vi "Main.vi"() -> ()   [LabVIEW 2017]
doc: "This Continuous Measurement sample project is based on the Queued Message Handler template.\n\nThe Event Handling Loop generates messages based on user interface actions.\n\nThe Message Handling Loop processes messages generated by the Event Handling Loop, or by other messages. There are also Acquisition and Logging message handling loop subVIs, and a chart updating loop."
uses:
  Settings/Settings.ctl
  Acquisition/Hardware Configuration.ctl
  Acquisition/Signal Type.ctl
  Logging/Logging Configuration.ctl
  controls/UI Data.ctl
  controls/UI State.ctl
  support/Message Queue/Enqueue Message (Single).vi
  support/Message Queue/Enqueue Message (Array).vi
  <vilib>/Utility/error.llb/Error Cluster From Error Code.vi
  <vilib>/ErrorRing/Error Ring.xnode
  Acquisition/Acquisition.lvlib
  Logging/Logging.lvlib
  Settings/Settings.lvlib
  support/User Event - Stop/User Event - Stop.lvlib
  support/Message Queue/Message Queue.lvlib
  Settings/Settings Dialog.vi
panel:
  out "Zero run":bool
  in  "Zero run?":bool
  out "Max writing time to a file [min]":dbl
  out "Elapsed time":timestamp
  out "Test time zero run [s]":dbl
  out "Test time [s]":dbl
  in  "Start":bool
  in  "Stop":bool
  in  "Settings":bool
  out "Status":string
  in  "Exit":bool
  out "Log File Offsite Path":path
  out "Project code":string
  out "Offsite storage?":bool
  out "Log File Path":path
  out "Data":waveform(dbl)[](graph)
  # "Continuous Measurement Data Logger"
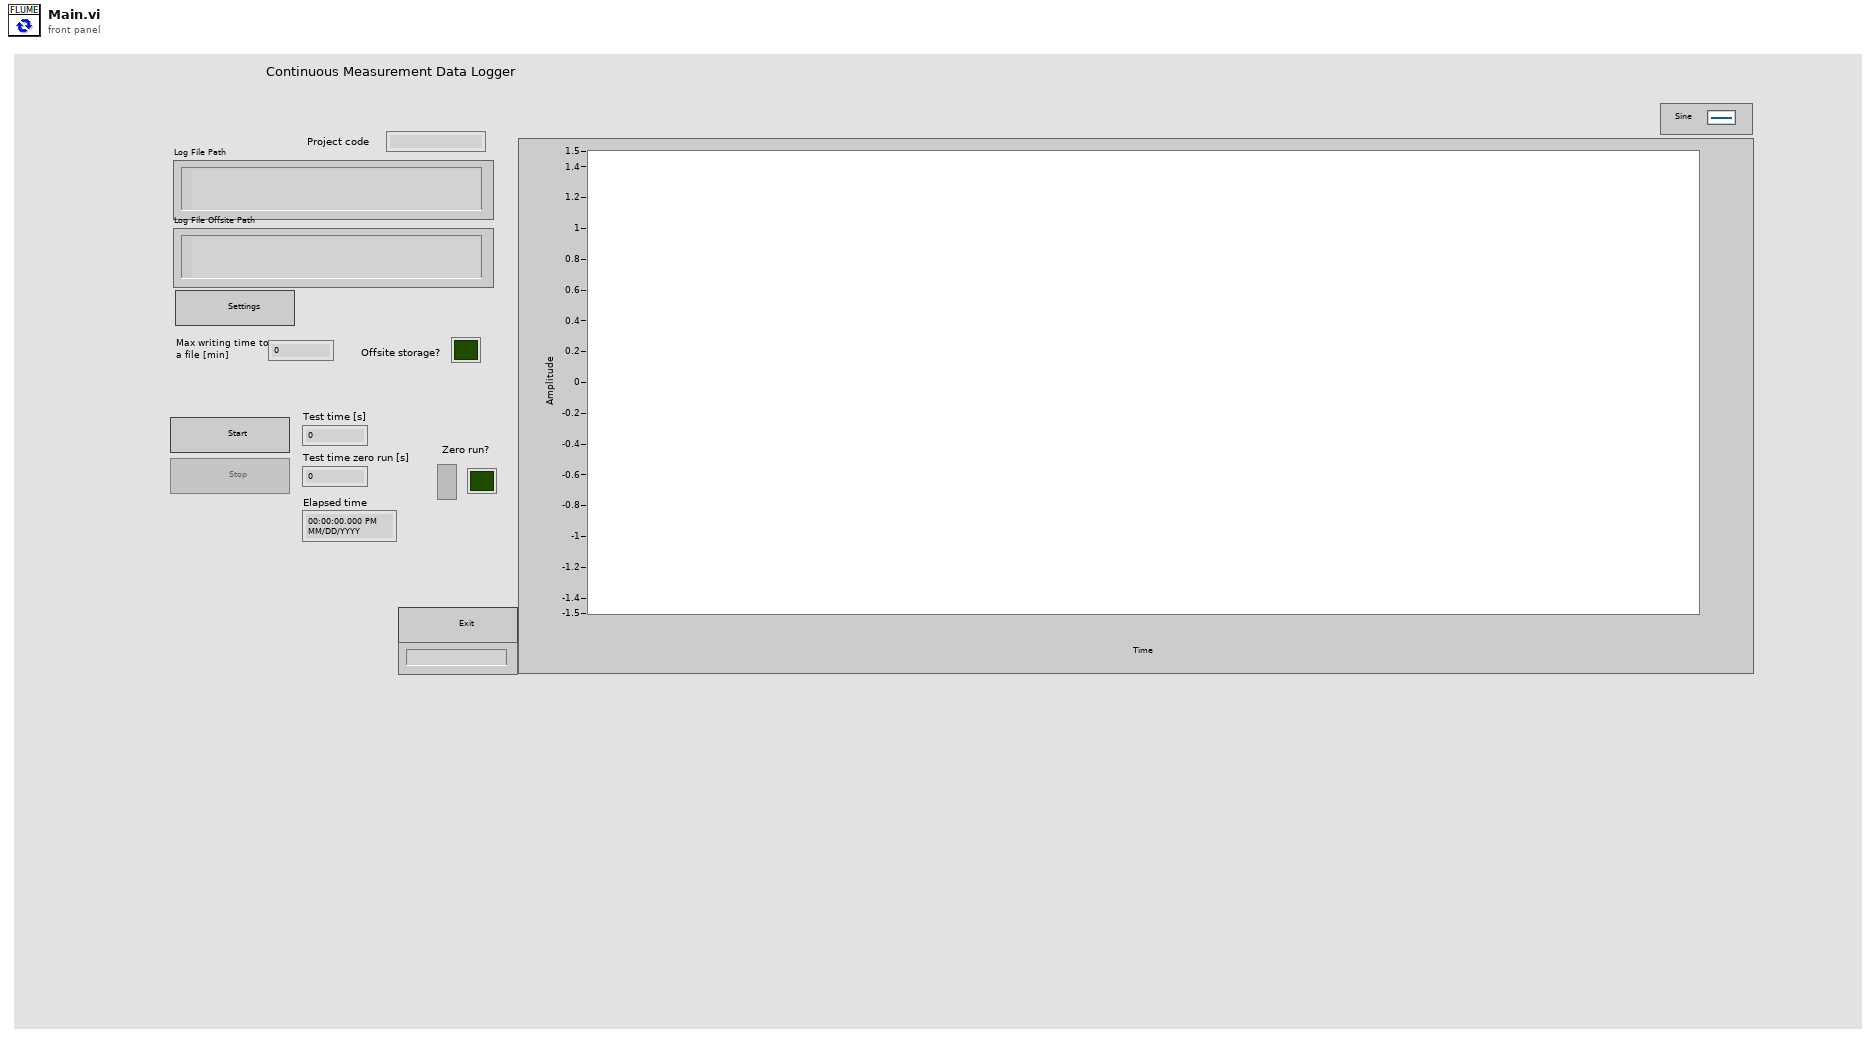
[diagram p1: front panel]
types:
  T1 = cluster{"Offsite storage?":bool, "Test time [s]":dbl, "Test time zero run [s] ":dbl, "Max writing time to a file [min]":dbl, "Zero run":bool}
  T2 = typedef "UI State.ctl" = enum16{"Idle", "Acquiring and Logging", "Waiting for Exit", "Waiting for Exit (Acq Stopped)", "Waiting for Exit (Log Stopped)", "Waiting for Stop", "Waiting for Stop (Acq Stopped)", "Waiting for Stop (Log Stopped)"}
  T3 = typedef "UI Data.ctl" = cluster{"Start Ref":refnum<vi>, "Stop Ref":refnum<vi>, "Settings Ref":refnum<vi>, "Exit Ref":refnum<vi>, "Status Ref":refnum<vi>, "Data Ref":refnum<vi>, "Zero run Ref":refnum<vi>}
  T4 = typedef "Settings.lvlib/Settings.ctl" = cluster{"Hardware Configuration":T5, "Logging Configuration":T7, "Timers":cluster{"Offsite storage?":bool, "Test time [s]":dbl, "Test time zero run [s] ":dbl, "Max writing time to a file [min]":dbl, "Zero run":bool}}
  T5 = typedef "Acquisition.lvlib/Hardware Configuration.ctl" = cluster{"HW Refnum <Replace Me>":string, "Signal Type <Replace Me>":T6}
  T6 = typedef "Acquisition.lvlib/Signal Type.ctl" = enum16{"Sine Wave", "Square with Noise"}
  T7 = typedef "Logging.lvlib/Logging Configuration.ctl" = cluster{"Log File Base Path":path, "TDMS File Reference":refnum<k34>, "Log File Offsite Path":path, "Project code":string, "Bin File Reference":refnum<file>}
  T8 = typedef "Message Queue.lvlib/All Message Queues.ctl" = cluster{"UI":refnum<queue>, "Acquisition":refnum<queue>, "Logging":refnum<queue>, "Bin Logging":refnum<queue>, "Time":refnum<queue>}
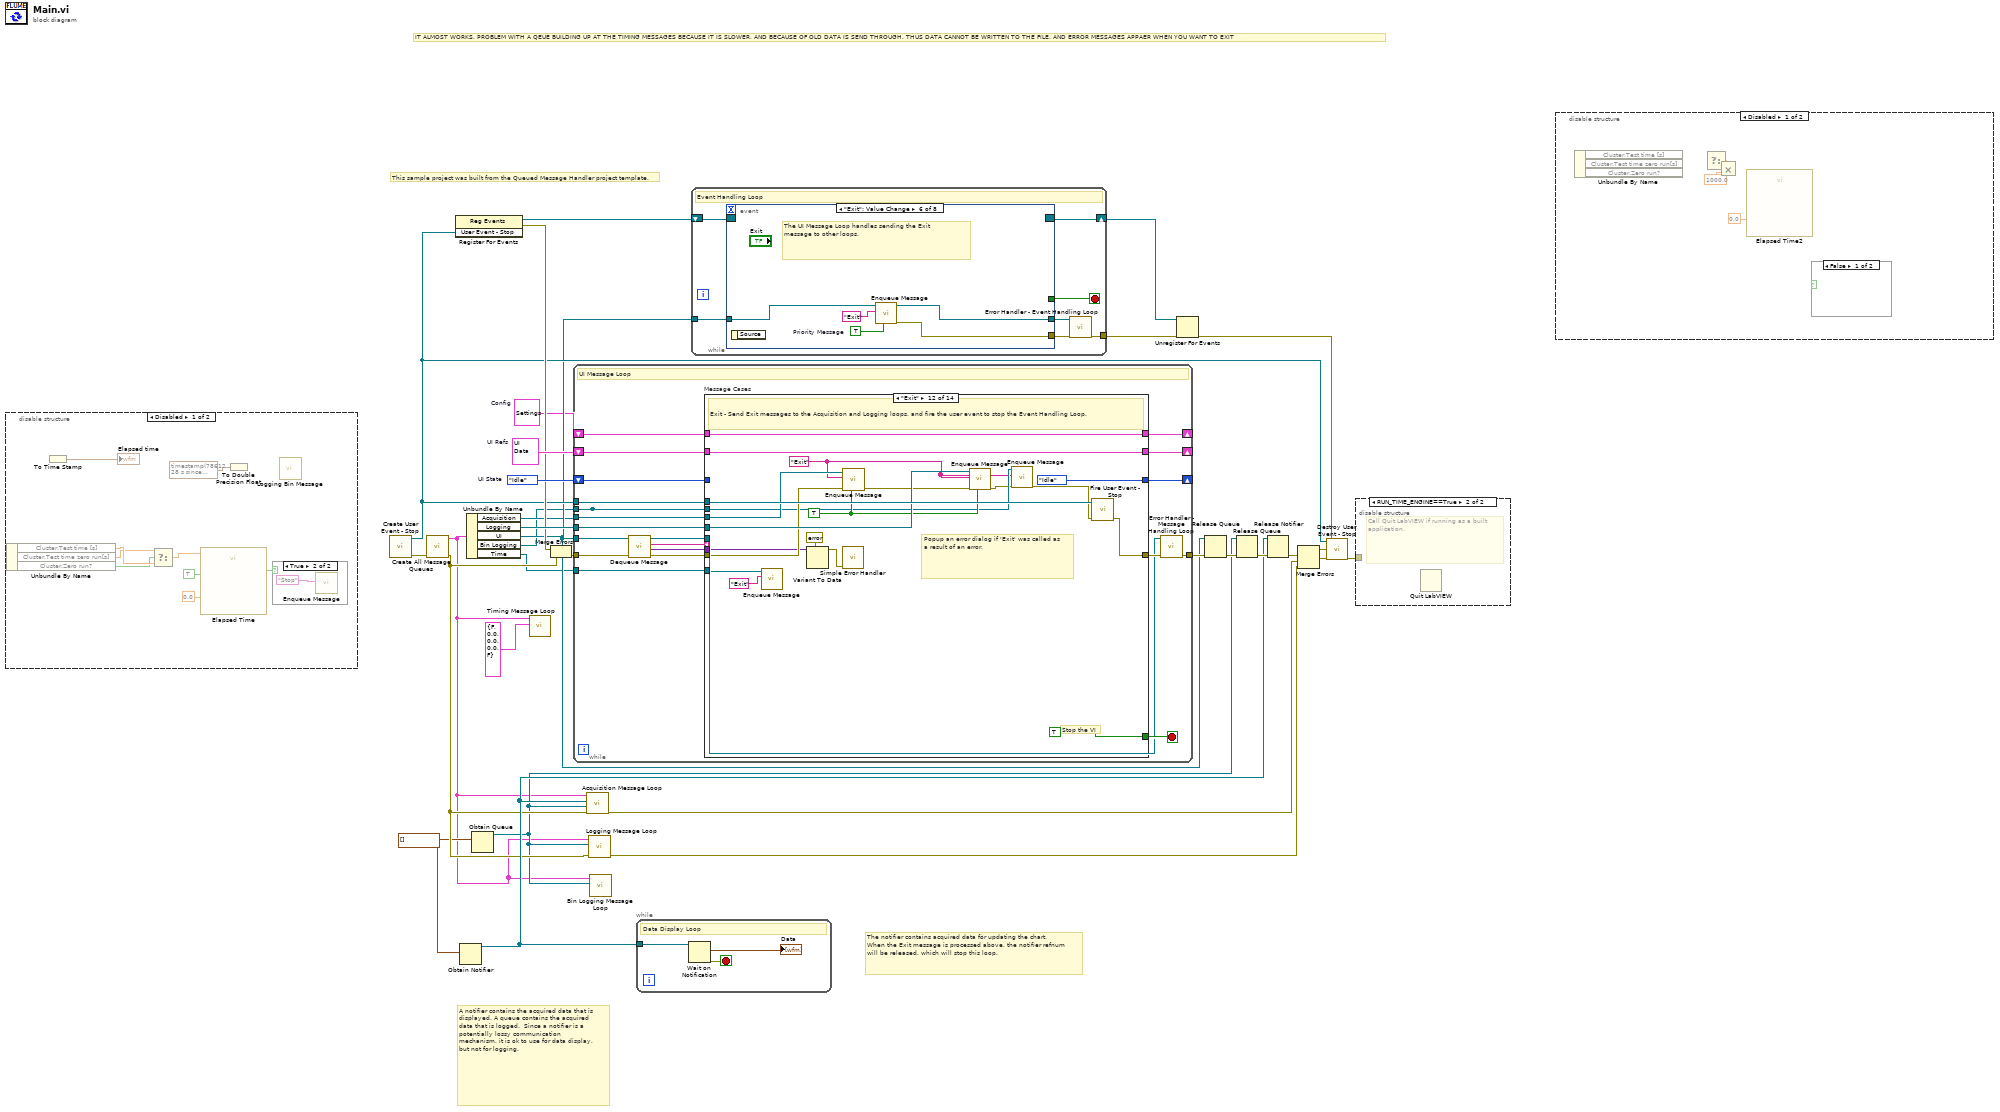
[diagram p0: block diagram]
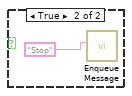
[diagram p2: hidden frame]
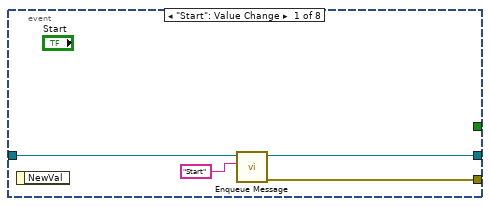
[diagram p7: hidden frame]
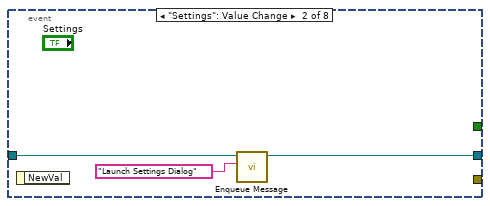
[diagram p8: hidden frame]
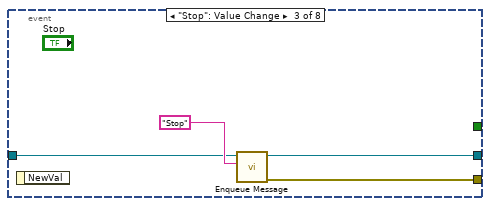
[diagram p9: hidden frame]
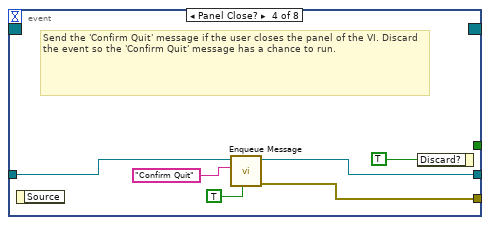
[diagram p10: hidden frame]
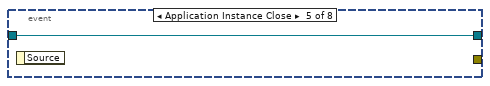
[diagram p11: hidden frame]
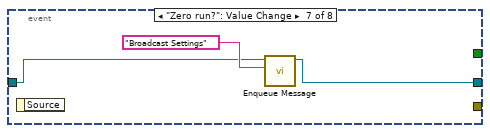
[diagram p12: hidden frame]
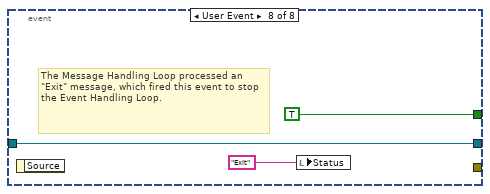
[diagram p13: hidden frame]
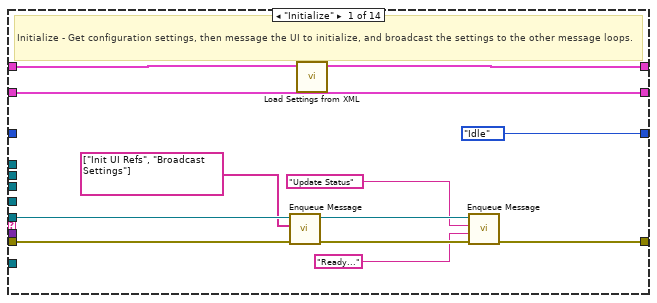
[diagram p14: hidden frame]
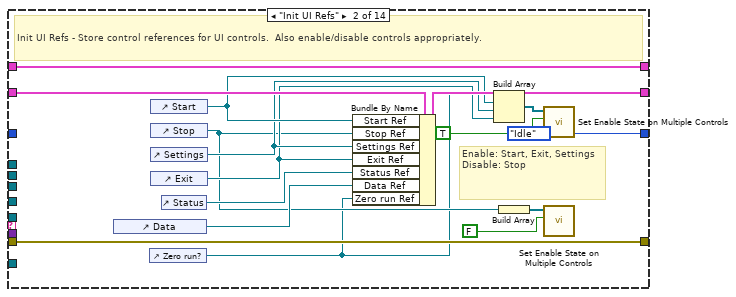
[diagram p15: hidden frame]
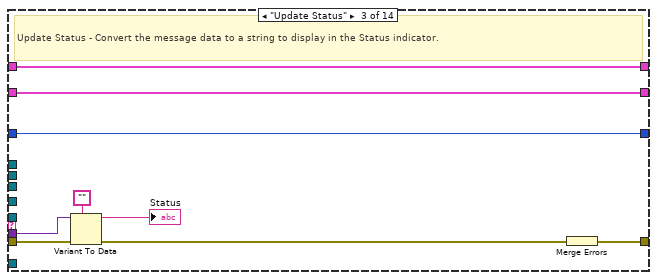
[diagram p16: hidden frame]
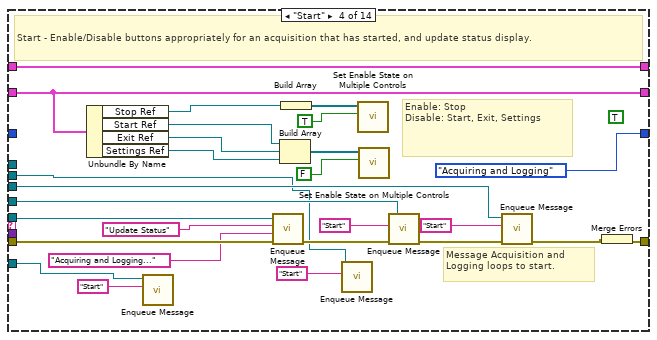
[diagram p17: hidden frame]
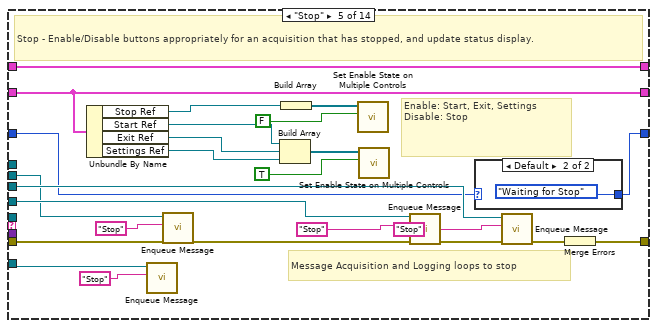
[diagram p18: hidden frame]
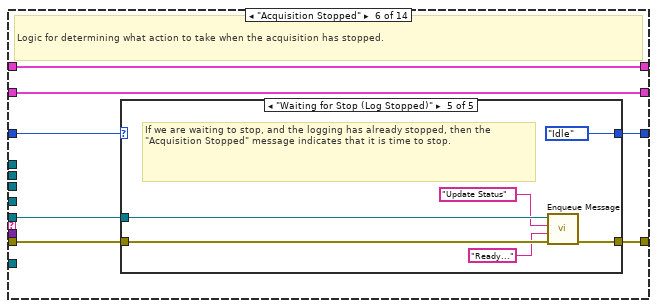
[diagram p20: hidden frame]
diagram:
  w23 = UI_State."Idle"  # UI State
  w7 = waveform(dbl)[] []
  w25 = T3 {"Start Ref"=refnum, "Stop Ref"=refnum, "Settings Ref"=refnum, "Exit Ref"=refnum, "Status Ref"=refnum, "Data Ref"=refnum, "Zero run Ref"=refnum}  # UI Refs
  w9 = T4 {"Hardware Configuration"={"HW Refnum <Replace Me>"="", "Signal Type <Replace Me>"=enum."Sine Wave"}, "Logging Configuration"={"Log File Base Path"=path "", "TDMS File Reference"=refnum, "Log File Offsite Path"=path "", "Project code"="", "Bin File Reference"=refnum}, "Timers"={"Offsite storage?"=FALSE, "Test time [s]"=10.0, "Test time zero run [s] "=180.0, "Max writing time to a file [min]"=30.0, "Zero run"=FALSE}}  # Config
  # "IT ALMOST WORKS, PROBLEM WITH A QEUE BUILDING UP AT THE TIMING MESSAGES BECAUSE IT IS SLOWER, AND BECAUSE OF OLD DATA IS SEND THROUGH, THUS DATA CANNOT BE WRITTEN TO THE FILE, AND ERROR MESSAGES APPAER WHEN YOU WANT TO EXIT"
  # "This sample project was built from the Queued Message Handler project template."
  # "A notifier contains the acquired data that is displayed. A queue contains the acquired data that is logged.  Since a notifier is a potentially lossy communication mechanism, it is ok to use for data display, but not for logging."
  # "The notifier contains acquired data for updating the chart. When the Exit message is processed above, the notifier refnum will be released, which will stop this loop."
  n1 = disable-structure shown="Disabled" {
    frame Disabled {
      n2 = Unbundle By Name() -> ("Cluster.Test time [s]"=w37:dbl, "Cluster.Test time zero run[s]"=w35:dbl, "Cluster.Zero run?"=w34:bool)  [unwired: 1 in]
      n3 = To Time Stamp() -> (0:→"Elapsed time":timestamp)  [unwired: 1 in]
      n4 = Select(t=w35, s=w34, f=w37) -> (s? t:f=w36:dbl)
      n5 = call "Elapsed Time"("Time Target (s)"=w36, "Auto Reset"=TRUE, "Set Start Time (s)"=0.0) -> ("Time has Elapsed"=w33:bool)  [unwired: 9 in, 7 out]
      n6 = To Double Precision Float(number=timestamp(7861228 s since 1904-01-01)) -> ()  [unwired: 1 out]
      n7 = case shown="True" w33 {
        frame False {
        }
        frame True {
          n8 = call-poly "Enqueue Message.vi"("Message"="Stop") -> ()  [unwired: 9 in, 2 out]
        }
      }
      n9 = call "Logging Bin Message.vi"() -> ()  [unwired: 11 in, 1 out]
    }
    frame Enabled {
    }
  }
  n10 = call "Create User Event - Stop.vi"() -> ("error out"=w27:errorcluster, "User Event - Stop"=w14:refnum<user-event>)  [unwired: 10 in]
  n11 = call "Create All Message Queues.vi"("error in (no error)"=w27) -> ("error out"=w8:errorcluster, "Message Queues out"=w2:T8)  [unwired: 9 in]
  n12 = register-events(w14) -> (reference out=w17:refnum<event-registration>, error out=w15:errorcluster)  [unwired: 2 in]
  n13 = Obtain Notifier(notification data type=w7) -> (notifier out=w10:refnum<notifier>)  [unwired: 3 in, 2 out]
  n14 = Unbundle By Name(w2) -> ("Acquisition"=w12:refnum<queue>, "Logging"=w24:refnum<queue>, "UI"=w13:refnum<queue>, "Bin Logging"=w5:refnum<queue>, "Time"=w1:refnum<queue>)
  n15 = Obtain Queue(element data type=w7) -> (queue out=w6:refnum<queue>)  [unwired: 4 in, 2 out]
  n16 = call "Timing Message Loop.vi"("Timers"=T1 {"Offsite storage?"=FALSE, "Test time [s]"=0.0, "Test time zero run [s] "=0.0, "Max writing time to a file [min]"=0.0, "Zero run"=FALSE}, "Message Queues"=w2) -> ()  [unwired: 9 in, 1 out]
  n17 = Merge Errors(w15, w8) -> (w16:errorcluster)
  n18 = while {
    tunnel: w13 -> [w46]
    tunnel: w14 -> [w59]
    shift-right: [w54] -> _
    shift-left: w9 -> [w42]
    shift-right: [w52] -> _
    shift-left: w25 -> [w53]
    tunnel: w12 -> [w51]
    tunnel: w24 -> [w45]
    shift-right: [w47] -> _
    shift-left: w23 -> [w48]
    tunnel: w16 -> [w58]
    tunnel: [w50] -> w30
    tunnel: w5 -> [w43]
    tunnel: [w43] -> _
    tunnel: w1 -> [w41]
    stop <- w60 stop-if-true
    # "UI Message Loop"
    n19 = call "Dequeue Message.vi"("error in (no error)"=w58, "Message Queue"=w46) -> ("error out"=w57:errorcluster, "Message Data"=w55:variant, "Message"=w56:string, "dup Message Queue"=w44:refnum<queue>)  [unwired: 6 in]
    n20 = case "Message Cases" shown="\"Exit\"" w56 {
      selector: w56 -> [_ _ _ _ _ _ _ _ _ _ _ _ _ w304]
      tunnel: w44 -> [w65 _ _ w103 _ w154 w179 _ w232 _ w254 _ _ _]
      tunnel: w57 -> [w64 w88 w96 w124 w147 w155 w180 w222 w234 w242 w253 w288 w302 _]
      tunnel: [w69 w88 w97 w105 w148 w152 w177 w226 w228 w245 w252 w295 w301 w303] -> w49
      tunnel: [_ _ _ _ _ _ _ _ _ _ _ TRUE _ _] -> w60
      tunnel: w55 -> [_ _ w95 _ _ _ _ _ _ w246 _ w286 _ _]
      tunnel: w59 -> [_ _ _ _ _ _ _ _ _ _ _ w296 _ _]
      tunnel: [w72 w75 w89 w101 w129 w151 w176 w205 w227 w241 w250 w284 w300 w307] -> w54
      tunnel: w42 -> [w61 w75 w89 w101 w129 w151 w176 w210 w235 w241 w250 w284 w300 w307]
      tunnel: w53 -> [w66 w87 w91 w121 w146 w157 w182 w221 w230 w249 w256 w294 w299 w306]
      tunnel: [w66 w84 w91 w121 w146 w157 w182 w221 w230 w249 w256 w294 w299 w306] -> w52
      tunnel: w51 -> [_ _ _ w104 w133 _ _ w220 _ _ _ w293 _ _]
      tunnel: w45 -> [_ _ _ w110 w136 _ _ w219 _ _ _ w292 _ _]
      tunnel: w48 -> [_ _ w90 _ w130 w156 w181 w218 w229 w244 w255 _ w298 w305]
      tunnel: [UI_State."Idle" ("UI State") UI_State."Idle" ("UI State") w90 UI_State."Acquiring and Logging" ("UI State") w131 w153 w178 w218 w229 w244 w251 UI_State."Idle" ("UI State") w298 w305] -> w47
      tunnel: w43 -> [_ _ _ w100 w127 _ _ w213 _ _ _ w283 _ _]
      tunnel: w41 -> [_ _ _ w98 w126 _ _ w209 _ _ _ w279 _ _]
      frame "Initialize" {
        # "Initialize - Get configuration settings, then message the UI to initialize, and broadcast the settings to the other message loops."
        n21 = call-poly "Enqueue Message.vi"("error in (no error)"=w64, "Message Array"=string[] ["Init UI Refs", "Broadcast Settings"], "Message Queue"=w65) -> ("error out"=w71:errorcluster, "dup Message Queue"=w70:refnum<queue>)  [unwired: 7 in]
        n22 = call "Load Settings from XML.vi"("Settings in"=w61) -> ("Settings out"=w72:T4)  [unwired: 9 in, 1 out]
        n23 = call-poly "Enqueue Message.vi"("error in (no error)"=w71, "Message Data"="Ready..." ("Ready..."), "Message"="Update Status", "Message Queue"=w70) -> ("error out"=w69:errorcluster)  [unwired: 6 in, 1 out]
      }
      frame "Init UI Refs" {
        # "Enable: Start, Exit, Settings\nDisable: Stop"
        # "Init UI Refs - Store control references for UI controls.  Also enable/disable controls appropriately."
        n24 = control-ref of="Data"() -> (w85:refnum<vi>)
        n25 = control-ref of="Zero run?"() -> (w73:refnum<vi>)
        n26 = control-ref of="Start"() -> (w79:refnum<vi>)
        n27 = control-ref of="Stop"() -> (w74:refnum<vi>)
        n28 = control-ref of="Settings"() -> (w78:refnum<vi>)
        n29 = control-ref of="Exit"() -> (w77:refnum<vi>)
        n30 = control-ref of="Status"() -> (w86:refnum<vi>)
        n31 = Bundle By Name(cluster=w87, "Start Ref"=w79, "Stop Ref"=w74, "Settings Ref"=w78, "Exit Ref"=w77, "Status Ref"=w86, "Data Ref"=w85, "Zero run Ref"=w73) -> (w84:T3)
        n32 = Build Array(w73, w79, w78, w77) -> (w82:refnum<vi>[])
        n33 = Build Array(w74) -> (w81:refnum<vi>[])
        n34 = call "Set Enable State on Multiple Controls.vi"("Enable?"=TRUE, "Controls"=w82) -> ()  [unwired: 10 in]
        n35 = call "Set Enable State on Multiple Controls.vi"("Enable?"=FALSE, "Controls"=w81) -> ()  [unwired: 10 in]
      }
      frame "Update Status" {
        # "Update Status - Convert the message data to a string to display in the Status indicator."
        n36 = Variant To Data(error in=w96, type="", Variant=w95) -> (data=→"Status":string, error out=w93:errorcluster)
        n37 = Merge Errors(w93) -> (w97:errorcluster)
      }
      frame "Start" {
        (unwired) TRUE ("Reset")
        # "Message Acquisition and Logging loops to start."
        # "Enable: Stop\nDisable: Start, Exit, Settings"
        # "Start - Enable/Disable buttons appropriately for an acquisition that has started, and update status display."
        n38 = Unbundle By Name(w121) -> ("Stop Ref"=w116:refnum<vi>, "Start Ref"=w115:refnum<vi>, "Exit Ref"=w114:refnum<vi>, "Settings Ref"=w113:refnum<vi>)
        n39 = call-poly "Enqueue Message.vi"("Message"="Start", "Message Queue"=w98) -> ()  [unwired: 8 in, 2 out]
        n40 = call-poly "Enqueue Message.vi"("error in (no error)"=w124, "Message Data"="Acquiring and Logging..." ("Acquiring and Logging..."), "Message"="Update Status", "Message Queue"=w103) -> ("error out"=w112:errorcluster)  [unwired: 6 in, 1 out]
        n41 = Build Array(w115, w114, w113) -> (w119:refnum<vi>[])
        n42 = Build Array(w116) -> (w118:refnum<vi>[])
        n43 = call-poly "Enqueue Message.vi"("Message"="Start", "Message Queue"=w100) -> ()  [unwired: 8 in, 2 out]
        n44 = call "Set Enable State on Multiple Controls.vi"("Enable?"=TRUE, "Controls"=w118) -> ()  [unwired: 10 in]
        n45 = call "Set Enable State on Multiple Controls.vi"("Enable?"=FALSE, "Controls"=w119) -> ()  [unwired: 10 in]
        n46 = call-poly "Enqueue Message.vi"("error in (no error)"=w112, "Message"="Start", "Message Queue"=w110) -> ("error out"=w107:errorcluster)  [unwired: 7 in, 1 out]
        n47 = call-poly "Enqueue Message.vi"("error in (no error)"=w107, "Message"="Start", "Message Queue"=w104) -> ("error out"=w106:errorcluster)  [unwired: 7 in, 1 out]
        n48 = Merge Errors(w106) -> (w105:errorcluster)
      }
      frame "Stop" {
        # "Message Acquisition and Logging loops to stop"
        # "Enable: Start, Exit, Settings\nDisable: Stop"
        # "Stop - Enable/Disable buttons appropriately for an acquisition that has stopped, and update status display."
        n49 = Unbundle By Name(w146) -> ("Stop Ref"=w141:refnum<vi>, "Start Ref"=w140:refnum<vi>, "Exit Ref"=w139:refnum<vi>, "Settings Ref"=w138:refnum<vi>)
        n50 = call-poly "Enqueue Message.vi"("Message"="Stop", "Message Queue"=w126) -> ()  [unwired: 8 in, 2 out]
        n51 = call-poly "Enqueue Message.vi"("Message"="Stop", "Message Queue"=w127) -> ()  [unwired: 8 in, 2 out]
        n52 = Build Array(w140, w139, w138) -> (w144:refnum<vi>[])
        n53 = Build Array(w141) -> (w143:refnum<vi>[])
        n54 = call "Set Enable State on Multiple Controls.vi"("Enable?"=FALSE, "Controls"=w143) -> ()  [unwired: 10 in]
        n55 = call "Set Enable State on Multiple Controls.vi"("Enable?"=TRUE, "Controls"=w144) -> ()  [unwired: 10 in]
        n56 = call-poly "Enqueue Message.vi"("error in (no error)"=w147, "Message"="Stop", "Message Queue"=w136) -> ("error out"=w135:errorcluster)  [unwired: 7 in, 1 out]
        n57 = case shown="Default" w130 {
          selector: w130 -> [w149 _]
          tunnel: [w149 UI_State."Waiting for Stop" ("UI State")] -> w131
          frame "Waiting for Exit" {
          }
          frame Default {
          }
        }
        n58 = call-poly "Enqueue Message.vi"("error in (no error)"=w135, "Message"="Stop", "Message Queue"=w133) -> ("error out"=w134:errorcluster)  [unwired: 7 in, 1 out]
        n59 = Merge Errors(w134) -> (w148:errorcluster)
      }
      frame "Acquisition Stopped" {
        # "Logic for determining what action to take when the acquisition has stopped."
        n60 = case shown="\"Waiting for Stop (Log Stopped)\"" w156 {
          selector: w156 -> [w159 _ _ _ _]
          tunnel: w155 -> [w158 w161 w163 w169 w175]
          tunnel: w154 -> [_ _ _ w167 w172]
          tunnel: [w159 UI_State."Waiting for Exit (Acq Stopped)" ("UI State") UI_State."Waiting for Stop (Acq Stopped)" ("UI State") UI_State."Idle" ("UI State") UI_State."Idle" ("UI State")] -> w153
          tunnel: [w158 w161 w163 w168 w173] -> w152
          frame Default {
          }
          frame "Waiting for Exit", "Waiting for Exit (Acq Stopped)" {
          }
          frame "Waiting for Stop", "Waiting for Stop (Acq Stopped)" {
          }
          frame "Waiting for Exit (Log Stopped)" {
            # "If we are waiting to exit, and the logging has already stopped, then the \"Acquisition Stopped\" message indicates that it is time to exit."
            n61 = call-poly "Enqueue Message.vi"("Priority Message? (F)"=TRUE, "error in (no error)"=w169, "Message"="Exit", "Message Queue"=w167) -> ("error out"=w168:errorcluster)  [unwired: 6 in, 1 out]
          }
          frame "Waiting for Stop (Log Stopped)" {
            # "If we are waiting to stop, and the logging has already stopped, then the \"Acquisition Stopped\" message indicates that it is time to stop."
            n62 = call-poly "Enqueue Message.vi"("error in (no error)"=w175, "Message Data"="Ready..." ("Ready..."), "Message"="Update Status", "Message Queue"=w172) -> ("error out"=w173:errorcluster)  [unwired: 6 in, 1 out]
          }
        }
      }
      frame "Logging Stopped" {
        # "Logic for determining what action to take when the logging has stopped."
        n63 = case shown="Default" w181 {
          selector: w181 -> [w184 _ _ _ _]
          tunnel: w180 -> [w183 w186 w188 w194 w197]
          tunnel: w179 -> [_ _ _ w192 w196]
          tunnel: [w184 UI_State."Waiting for Exit (Log Stopped)" ("UI State") UI_State."Waiting for Stop (Log Stopped)" ("UI State") UI_State."Idle" ("UI State") UI_State."Idle" ("UI State")] -> w178
          tunnel: [w183 w186 w188 w193 w195] -> w177
          frame Default {
          }
          frame "Waiting for Exit", "Waiting for Exit (Log Stopped)" {
          }
          frame "Waiting for Stop", "Waiting for Stop (Log Stopped)" {
          }
          frame "Waiting for Exit (Acq Stopped)" {
            # "If we are waiting to exit, and the acquisition has already stopped, then the \"Logging Stopped\" message indicates that it is time to exit."
            n64 = call-poly "Enqueue Message.vi"("Priority Message? (F)"=TRUE, "error in (no error)"=w194, "Message"="Exit", "Message Queue"=w192) -> ("error out"=w193:errorcluster)  [unwired: 6 in, 1 out]
          }
          frame "Waiting for Stop (Acq Stopped)" {
            # "If we are waiting to stop, and the acquisition has already stopped, then the \"Logging Stopped\" message indicates that it is time to stop."
            n65 = call-poly "Enqueue Message.vi"("error in (no error)"=w197, "Message Data"="Ready..." ("Ready..."), "Message"="Update Status", "Message Queue"=w196) -> ("error out"=w195:errorcluster)  [unwired: 6 in, 1 out]
          }
        }
      }
      frame "Broadcast settings" {
        w208 = "Update Settings" ("Message")
        # "Broadcast settings - Send the 'Update Settings' message to the Logging and Acquisition message loops."
        n66 = Unbundle By Name(w210) -> ("Hardware Configuration"=w224:T5, "Logging Configuration"=w212:T7, "Timers"=w207:T1)
        n67 = Unbundle By Name(w212) -> ("Log File Base Path"=→"Log File Path":path, "Log File Offsite Path"=→"Log File Offsite Path":path, "Project code"=→"Project code":string)
        n68 = Bundle By Name(cluster=w210, "Timers.Zero run"="Zero run?") -> (w205:T4)
        n69 = Unbundle By Name(w207) -> ("Max writing time to a file [min]"=→"Max writing time to a file [min]":dbl, "Offsite storage?"=→"Offsite storage?":bool, "Test time [s]"=→"Test time [s]":dbl, "Test time zero run [s]"=→"Test time zero run [s]":dbl)
        n70 = Unbundle By Name(w205) -> ("Timers"=w204:T1)
        n71 = call-poly "Enqueue Message.vi"("Message Data"=w224, "Message"=w208, "Message Queue"=w220) -> ("error out"=w225:errorcluster)  [unwired: 7 in, 1 out]
        n72 = call-poly "Enqueue Message.vi"("Message Data"=w204, "Message"=w208, "Message Queue"=w209) -> ("error out"=w203:errorcluster)  [unwired: 7 in, 1 out]
        n73 = call-poly "Enqueue Message.vi"("Message Data"=w212, "Message"=w208, "Message Queue"=w213) -> ()  [unwired: 7 in, 2 out]
        n74 = call-poly "Enqueue Message.vi"("error in (no error)"=w225, "Message Data"=w212, "Message"=w208, "Message Queue"=w219) -> ("error out"=w223:errorcluster)  [unwired: 6 in, 1 out]
        n75 = Merge Errors(w223, w222, w203) -> (w226:errorcluster)
        "Zero run" <- "Zero run?"
      }
      frame "Launch Settings Dialog" {
        # "Launch Settings Dialog - Launch the Settings Dialog when the user clicks the 'Settings' button."
        n76 = call-by-ref "?"("error in (no error)"=w234, "Settings in"=w235) -> ("error out"=w231:errorcluster, "Cancelled?"=w233:bool, "Settings out"=w227:T4)  [unwired: 8 in, 3 out]
        n77 = case shown="False" w233 {
          tunnel: w232 -> [w239 _]
          tunnel: w231 -> [w238 w240]
          tunnel: [w237 w240] -> w228
          frame False {
            n78 = call-poly "Enqueue Message.vi"("error in (no error)"=w238, "Message"="Broadcast Settings", "Message Queue"=w239) -> ("error out"=w237:errorcluster)  [unwired: 7 in, 1 out]
          }
          frame True {
          }
        }
      }
      frame "Error" {
        # "Error - Display an error dialog. This message is sent by the \"Error Handler\" VIs at the end of other loops in this application."
        n79 = Variant To Data(error in=w242, type=errorcluster {"status"=FALSE, "code"=0, "source"=""} ("error constant"), Variant=w246) -> (data=w243:errorcluster, error out=w247:errorcluster)
        n80 = call <vilib>:"Simple Error Handler.vi"("error in (no error)"=w243) -> ()  [unwired: 4 in, 5 out]
        n81 = Merge Errors(w247) -> (w245:errorcluster)
      }
      frame "Confirm Quit" {
        # "Confirm Quit - Message that can confirm whether or not the user wants to exit the application."
        n82 = case shown="\"Acquiring and Logging\"" w255 {
          tunnel: w254 -> [w262 w266]
          tunnel: w253 -> [w261 w265]
          tunnel: [w260 w264] -> w252
          tunnel: [UI_State."Idle" ("UI State") w263] -> w251
          frame Default {
            # "If 'Confirm Quit' comes in while the system is idle, there is no need for a confirmation message."
            n83 = call-poly "Enqueue Message.vi"("Priority Message? (F)"=TRUE, "error in (no error)"=w261, "Message"="Exit", "Message Queue"=w262) -> ("error out"=w260:errorcluster)  [unwired: 6 in, 1 out]
          }
          frame "Acquiring and Logging" {
            n84 = Two Button Dialog(message="Are you sure you want to quit while the acquisition is running?" ("Confirm Quit Message"), 1:"No" ("No"), 2:"Yes" ("Yes")) -> (T button?=w267:bool)
            n85 = case shown="True" w267 {
              tunnel: w266 -> [_ w276]
              tunnel: w265 -> [w272 w277]
              tunnel: [w272 w275] -> w264
              tunnel: [UI_State."Acquiring and Logging" ("UI State") UI_State."Waiting for Exit" ("UI State")] -> w263
              frame False {
                # "User did not want to quit."
              }
              frame True {
                n86 = call-poly "Enqueue Message.vi"("error in (no error)"=w277, "Message"="Stop", "Message Queue"=w276) -> ("error out"=w275:errorcluster)  [unwired: 7 in, 1 out]
              }
            }
          }
        }
      }
      frame "Exit" {
        w289 = TRUE ("Priority Message? (F)")
        w282 = "Exit" ("Message")
        # "Popup an error dialog if 'Exit' was called as a result of an error."
        # "Stop the VI"
        # "Exit - Send Exit messages to the Acquisition and Logging loops, and fire the user event to stop the Event Handling Loop."
        n87 = call-poly "Enqueue Message.vi"("Message"="Exit", "Message Queue"=w279) -> ()  [unwired: 8 in, 2 out]
        n88 = Variant To Data(type=errorcluster {"status"=FALSE, "code"=0, "source"=""} ("error constant"), Variant=w286) -> (data=w285:errorcluster)  [unwired: 1 in, 1 out]
        n89 = call <vilib>:"Simple Error Handler.vi"("error in (no error)"=w285) -> ()  [unwired: 4 in, 5 out]
        n90 = call-poly "Enqueue Message.vi"("Priority Message? (F)"=w289, "error in (no error)"=w288, "Message"=w282, "Message Queue"=w293) -> ("error out"=w290:errorcluster)  [unwired: 6 in, 1 out]
        n91 = call-poly "Enqueue Message.vi"("Priority Message? (F)"=w289, "error in (no error)"=w290, "Message"=w282, "Message Queue"=w292) -> ("error out"=w281:errorcluster)  [unwired: 6 in, 1 out]
        n92 = call-poly "Enqueue Message.vi"("error in (no error)"=w281, "Message"=w282, "Message Queue"=w283) -> ("error out"=w280:errorcluster)  [unwired: 7 in, 1 out]
        n93 = call "Fire User Event - Stop.vi"("error in (no error)"=w280, "User Event - Stop"=w296) -> ("error out"=w295:errorcluster)  [unwired: 9 in]
      }
      frame "---Copy This Frame---" {
        (unwired) FALSE ("Time has Elapsed")
        # "Duplicate this frame when creating new messages.  Change this comment in the duplicated frame to describe this message."
        n94 = Merge Errors(w302) -> (w301:errorcluster)
      }
      frame Default {
        # "'Default' case only runs if there is a message that isn't defined in any of the other cases.  Output a programming error."
        n95 = xnode "Error Ring"("parameter 0"=w304) -> ("error out"=w303:errorcluster)
      }
    }
    n96 = call "Error Handler - Message Handling Loop.vi"("error in (no error)"=w49, "Message Queue"=w44) -> ("dup error in"=w50:errorcluster)  [unwired: 8 in, 1 out]
  }
  n97 = call "Acquisition Message Loop.vi"("error in (no error)"=w8, "Data Queue"=w6, "Data Notifier"=w10, "Message Queues"=w2) -> ("error out"=w28:errorcluster)  [unwired: 7 in]
  n98 = call "Logging Message Loop.vi"("error in (no error)"=w8, "Data Queue"=w6, "Message Queues"=w2) -> ("error out"=w4:errorcluster)  [unwired: 8 in]
  n99 = call "Bin Logging Message Loop.vi"("Data Queue"=w6, "Message Queues"=w2) -> ()  [unwired: 9 in, 1 out]
  n100 = while "Data Display Loop" {
    tunnel: w10 -> [w317]
    stop <- w316 stop-if-true
    # "Data Display Loop"
    n101 = Wait on Notification(notifier=w317) -> (notification=→"Data":waveform(dbl)[], error out=w316:errorcluster)  [unwired: 3 in, 2 out]
  }
  n102 = while {
    tunnel: w13 -> [w323]
    tunnel: [w320] -> w29
    shift-right: [w322] -> w26
    shift-left: w17 -> [w324]
    stop <- w321 stop-if-true
    # "Event Handling Loop"
    n103 = event shown="[5] \"Exit\": Value Change" {
      selector: w324 -> [_ _ _ _ _ _ _ _]
      dyn-events: [_ _ _ _ _ _ _ _] -> w322
      timeout: _ -> [_ _ _ _ _ _ _ _]
      tunnel: [_ _ _ _ _ _ _ TRUE ("Discard?")] -> w321
      tunnel: w323 -> [w328 w330 w334 w339 w342 w344 w349 w351]
      tunnel: [w326 _ w333 w337 _ w347 _ _] -> w319
      tunnel: [w325 w329 w332 w338 w342 w343 w348 w351] -> w318
      event "Start": Value Change {
        n104 = event-data() -> ()  [unwired: 1 in, 1 out]
        n105 = call-poly "Enqueue Message.vi"("Message"="Start", "Message Queue"=w328) -> ("error out"=w326:errorcluster, "dup Message Queue"=w325:refnum<queue>)  [unwired: 8 in]
      }
      event "Settings": Value Change {
        n106 = event-data() -> ()  [unwired: 1 in, 1 out]
        n107 = call-poly "Enqueue Message.vi"("Message"="Launch Settings Dialog", "Message Queue"=w330) -> ("dup Message Queue"=w329:refnum<queue>)  [unwired: 8 in, 1 out]
      }
      event "Stop": Value Change {
        n108 = event-data() -> ()  [unwired: 1 in, 1 out]
        n109 = call-poly "Enqueue Message.vi"("Message"="Stop", "Message Queue"=w334) -> ("error out"=w333:errorcluster, "dup Message Queue"=w332:refnum<queue>)  [unwired: 8 in]
      }
      event Panel Close? {
        # "Send the 'Confirm Quit' message if the user closes the panel of the VI. Discard the event so the 'Confirm Quit' message has a chance to run."
        n110 = event-data() -> ()  [unwired: 1 in, 1 out]
        n111 = call-poly "Enqueue Message.vi"("Priority Message? (F)"=TRUE, "Message"="Confirm Quit", "Message Queue"=w339) -> ("error out"=w337:errorcluster, "dup Message Queue"=w338:refnum<queue>)  [unwired: 7 in]
        n112 = event-data("Discard?"=TRUE) -> ()  [unwired: 1 in, 1 out]
      }
      event Application Instance Close {
        n113 = event-data() -> ()  [unwired: 1 in, 1 out]
      }
      event "Exit": Value Change {
        w345 = TRUE  # Priority Message
        # "The UI Message Loop handles sending the Exit message to other loops."
        n114 = event-data() -> ()  [unwired: 1 in, 1 out]
        n115 = call-poly "Enqueue Message.vi"("Priority Message? (F)"=w345, "Message"="Exit", "Message Queue"=w344) -> ("error out"=w347:errorcluster, "dup Message Queue"=w343:refnum<queue>)  [unwired: 7 in]
      }
      event "Zero run?": Value Change {
        n116 = event-data() -> ()  [unwired: 1 in, 1 out]
        n117 = call-poly "Enqueue Message.vi"("Message"="Broadcast Settings", "Message Queue"=w349) -> ("dup Message Queue"=w348:refnum<queue>)  [unwired: 8 in, 1 out]
      }
      event User Event {
        # "The Message Handling Loop processed an \"Exit\" message, which fired this event to stop the Event Handling Loop."
        n118 = event-data() -> ()  [unwired: 1 in, 1 out]
        n119 = local write "Status"("Exit" ("Exit String")) -> ()
      }
    }
    n120 = call "Error Handler - Event Handling Loop.vi"("error in (no error)"=w319, "Message Queue"=w318) -> ("dup error in"=w320:errorcluster)  [unwired: 8 in, 1 out]
  }
  n121 = Unregister For Events(event registration refnum=w26, error in=w29) -> (error out=w11:errorcluster)
  n122 = Release Queue(queue=w13, error in (no error)=w30) -> (error out=w20:errorcluster)  [unwired: 1 in, 2 out]
  n123 = Release Queue(queue=w6, error in (no error)=w20) -> (error out=w19:errorcluster)  [unwired: 1 in, 2 out]
  n124 = Release Notifier(notifier=w10, error in (no error)=w19) -> (error out=w18:errorcluster)  [unwired: 1 in, 2 out]
  n125 = Merge Errors(w11, w18, w28, w4) -> (w22:errorcluster)
  n126 = call "Destroy User Event - Stop.vi"("error in (no error)"=w22, "User Event - Stop"=w14) -> ("error out"=w21:errorcluster)  [unwired: 9 in]
  n127 = disable-structure shown="RUN_TIME_ENGINE==True" {
    disable-tunnel: w21 -> [_ _]
    frame condition #0 (active) {
    }
    frame condition #1 {
      # "Call Quit LabVIEW if running as a built application."
      n128 = Quit LabVIEW() -> ()  [unwired: 1 in]
    }
  }
  n129 = disable-structure shown="Disabled" {
    frame Disabled {
      n130 = Unbundle By Name() -> ()  [unwired: 1 in, 3 out]
      n131 = Select() -> (s? t:f=w356:dbl)  [unwired: 3 in]
      n132 = Multiply(x=w356, y=1000.0) -> ()  [unwired: 1 out]
      n133 = call "Elapsed Time2"("Set Start Time (s)"=0.0) -> ()  [unwired: 11 in, 8 out]
      n134 = case shown="False" {
        selector: _ -> [_ _]
        frame False {
        }
        frame True {
          n135 = call-poly "Enqueue Message.vi"("Message"="Stop") -> ()  [unwired: 9 in, 2 out]
        }
      }
    }
    frame Enabled {
    }
  }
